vi "catalog.create_dataset.vi"(8 "error in":errorcluster, 10 "name":string, 11 "Nominal Client in":refnum<class "Nominal Client.lvclass">) -> (0 "error out":errorcluster, 2 "Dataset":refnum<class "dataset.lvclass">, 3 "Nominal Client out":refnum<class "Nominal Client.lvclass">)   [LabVIEW 2020, in "Nominal Client.lvclass"]
doc: "Create a dataset"
uses:
  Nominal Client.lvclass
  datasources/dataset/dataset.lvclass
  Nominal Client.lvclass/Nominal Client.ctl
  trace.payload_received.vi
  error.vi
  trace.payload_sent.vi
  create.authorization_header.vi
  trace.calling_method.vi
  error.vi/859f8e04-e495-489b-b5b4-7ac163f56130.vi
  <vilib>/JDP Science/JDP Science Common Utilities/Trim Whitespace__JDP.vi
  <vilib>/AdvancedString/1D String Array to Delimited String.vi
  api_token.get.vi
  <vilib>/Utility/libraryn.llb/Get File Extension.vi
  log_file.write.vi
  submodules/reqwest-labview/lv-src/reqwest/post.vi
  <vilib>/JDP Science/JSONtext/Get all Object Items.vi
  <vilib>/Utility/error.llb/Error Cluster From Error Code.vi
  <vilib>/JDP Science/JSONtext/JSON text to Variant.vi
  <vilib>/JDP Science/JSONtext/LVClass Serializer/JSONtext LVClass Serializer.lvclass
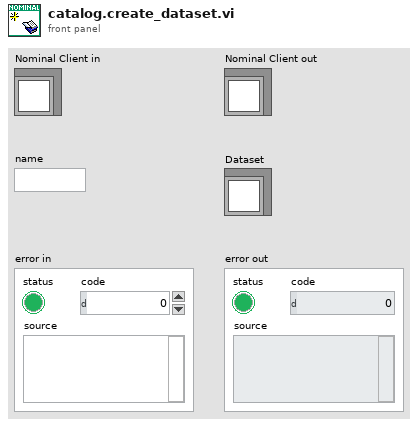
[diagram p1: front panel]
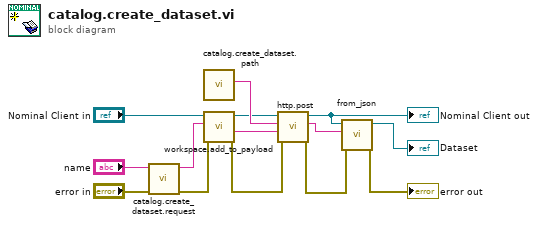
[diagram p0: block diagram]
diagram:
  n1 = call "catalog.create_dataset.request.vi"("error in"="error in", "name"="name") -> ("error out"=w2:errorcluster, "request"=w6:string)  [unwired: 8 in]
  n2 = call "catalog.create_dataset.path.vi"() -> ("path"=w14:string)  [unwired: 11 in]
  n3 = call "workspace.add_to_payload.vi"("error in"=w2, "JSON payload in"=w6, "Nominal Client in"="Nominal Client in") -> ("error out"=w1:errorcluster, "JSON payload out"=w5:string, "Nominal Client out"=w3:refnum<class "Nominal Client.lvclass">)  [unwired: 6 in]
  n4 = call "http.post.vi"("error in"=w1, "Request body"=w5, "Path"=w14, "Nominal Client in"=w3) -> ("error out"=w11:errorcluster, "Response"=w7:string, "Nominal Client out"=w8:refnum<class "Nominal Client.lvclass">)  [unwired: 5 in]
  "Nominal Client out" <- w8
  n5 = call "from_json.vi"("error in"=w11, "dataset JSON"=w7, "Client"=w8) -> ("error out"=→"error out":errorcluster, "Dataset"=→"Dataset":refnum<class "dataset.lvclass">)  [unwired: 7 in]
